vi "Digital Close.vi"(8 "error in (no error)":errorcluster, 11 "Semiconductor Module Context":T1) -> (0 "error out":errorcluster)   [LabVIEW 2014]
uses:
  <vilib>/NI_TestStand_SemiconductorModule/NI_TestStand_Semiconductor_Module.lvlibp/PinMap/General/SemiconductorModuleContext.ctl
  <vilib>/NI_TestStand_SemiconductorModule/NI_TestStand_Semiconductor_Module.lvlibp
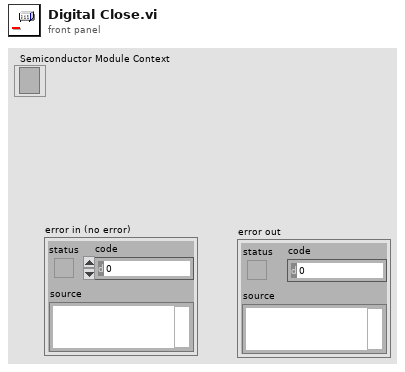
[diagram p1: front panel]
types:
  T1 = typedef "NI_TestStand_Semiconductor_Module.lvlibp/SemiconductorModuleContext.ctl" = refnum<k7>
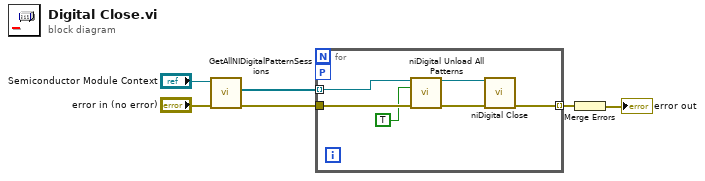
[diagram p0: block diagram]
diagram:
  n1 = call <vilib>:"GetAllNIDigitalPatternSessions.vi"("error in (no error)"="error in (no error)", "Semiconductor Module Context"="Semiconductor Module Context") -> ("error out"=w6:errorcluster, "Instrument Sessions"=w5:refnum<k15>[])  [unwired: 7 in, 1 out]
  n2 = for {
    tunnel: w5 -> [w9] mode=indexing
    tunnel: w6 -> [w8]
    tunnel: [w12] -> w2 mode=indexing
    workers-P: _ -> [_]
    n3 = call <instrlib>:"niDigital Unload All Patterns.vi"("instrument handle"=w9, "unload keep alive pattern (F)"=TRUE, "error in"=w8) -> ("instrument handle out"=w10:refnum<k15>, "error out"=w11:errorcluster)  [unwired: 11 in]
    n4 = call <instrlib>:"niDigital Close.vi"("instrument handle"=w10, "error in"=w11) -> ("error out"=w12:errorcluster)  [unwired: 13 in]
  }
  n5 = Merge Errors(w2) -> (→"error out":errorcluster)
